vi "PivotHoldSide.vi"(10 "CurrEnc":dbl, 11 "FirstTime?":bool) -> (3 "MtrPwrOut":dbl)   [LabVIEW 2017]
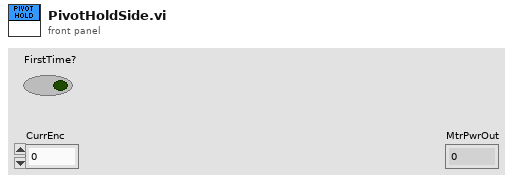
[diagram p1: front panel]
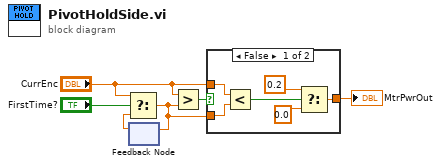
[diagram p0: block diagram]
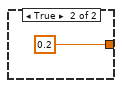
[diagram p2: hidden frame]
diagram:
  n1 = feedback #1() -> (w6:dbl)  [unwired: 1 in]
  n2 = Select(t="CurrEnc", s="FirstTime?", f=w6) -> (s? t:f=w2:dbl)
  n3 = feedback-in #1(w2) -> ()
  n4 = Greater?(x="CurrEnc", y=w2) -> (0:w4:bool)
  n5 = case shown="False" w4 {
    tunnel: "CurrEnc" -> [w10 _]
    tunnel: w2 -> [w9 _]
    tunnel: [w7 0.2] -> w1
    frame False {
      n6 = Less?(x=w10, y=w9) -> (x < y?=w8:bool)
      n7 = Select(t=0.2, s=w8, f=0.0) -> (s? t:f=w7:dbl)
    }
    frame True {
    }
  }
  "MtrPwrOut" <- w1
